vi "Draw_Grid.vi"(6 "Grid Color":u32(colorbox)=16711680, 8 "error in (no error)":errorcluster, 10 "Grid_Size":i32, 11 "Image_In":T1) -> (0 "error out":errorcluster, 3 "Image_Out":T1)   [LabVIEW 2020]
uses:
  <vilib>/vision/Image Controls.llb/IMAQ Image.ctl
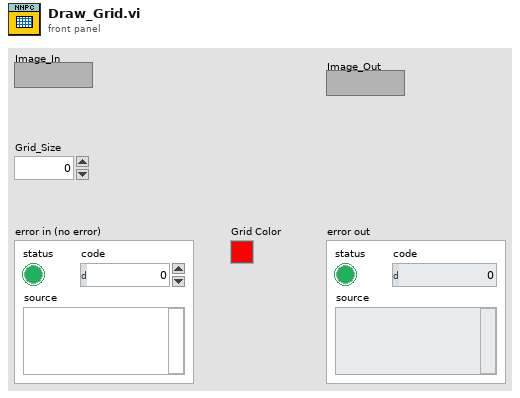
[diagram p1: front panel]
types:
  T1 = typedef "IMAQ Image.ctl" = refnum<image>
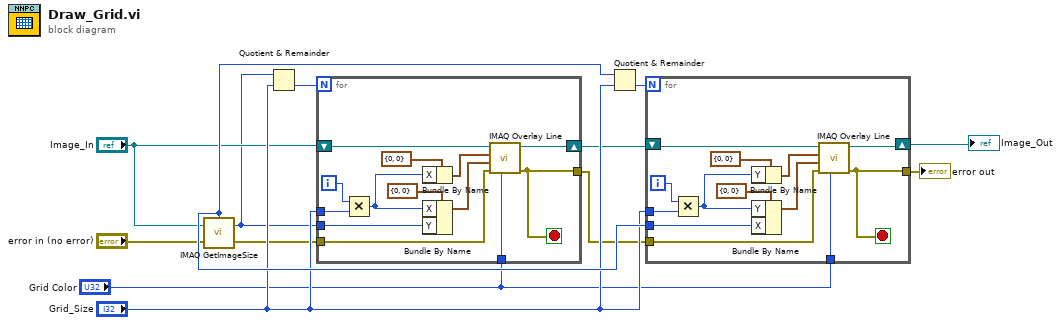
[diagram p0: block diagram]
diagram:
  n1 = call "IMAQ GetImageSize"("Image"="Image_In", "error in (no error)"="error in (no error)") -> ("Y Resolution"=w5:i32, "X Resolution"=w12:i32, "error out"=w4:errorcluster)  [unwired: 2 in]
  n2 = Quotient & Remainder(x=w5, y="Grid_Size") -> (floor(x/y)=w6:i32)  [unwired: 1 out]
  n3 = for {
    N: w6 -> [_]
    tunnel: w5 -> [w22]
    tunnel: w4 -> [w21]
    tunnel: "Grid_Size" -> [w20]
    tunnel: [w16] -> w9
    shift-right: [w15] -> w8
    shift-left: "Image_In" -> [w17]
    tunnel: "Grid Color" -> [w14]
    i -> [w19]
    stop <- w16 stop-if-true
    n4 = Multiply(x=w19, y=w20) -> (x*y=w18:i32)
    n5 = Bundle By Name(cluster=cluster{"X":i32, "Y":i32} {"X"=0, "Y"=0} ("Start Point"), "X"=w18) -> (w25:cluster{"X":i32, "Y":i32})
    n6 = Bundle By Name(cluster=cluster{"X":i32, "Y":i32} {"X"=0, "Y"=0} ("Start Point"), "X"=w18, "Y"=w22) -> (w23:cluster{"X":i32, "Y":i32})
    n7 = call "IMAQ Overlay Line"("Color"=w14, "error in (no error)"=w21, "End Point"=w23, "Start Point"=w25, "Image"=w17) -> ("error out"=w16:errorcluster, "Image Out"=w15:T1)  [unwired: 5 in]
  }
  n8 = Quotient & Remainder(x=w12, y="Grid_Size") -> (floor(x/y)=w10:i32)  [unwired: 1 out]
  n9 = for {
    N: w10 -> [_]
    tunnel: w12 -> [w29]
    tunnel: w9 -> [w35]
    tunnel: "Grid_Size" -> [w34]
    tunnel: [w30] -> w2
    shift-right: [w28] -> w13
    shift-left: w8 -> [w31]
    tunnel: "Grid Color" -> [w27]
    i -> [w33]
    stop <- w30 stop-if-true
    n10 = Multiply(x=w33, y=w34) -> (x*y=w32:i32)
    n11 = Bundle By Name(cluster=cluster{"X":i32, "Y":i32} {"X"=0, "Y"=0} ("Start Point"), "Y"=w32) -> (w38:cluster{"X":i32, "Y":i32})
    n12 = Bundle By Name(cluster=cluster{"X":i32, "Y":i32} {"X"=0, "Y"=0} ("Start Point"), "Y"=w32, "X"=w29) -> (w36:cluster{"X":i32, "Y":i32})
    n13 = call "IMAQ Overlay Line"("Color"=w27, "error in (no error)"=w35, "End Point"=w36, "Start Point"=w38, "Image"=w31) -> ("error out"=w30:errorcluster, "Image Out"=w28:T1)  [unwired: 5 in]
  }
  "Image_Out" <- w13
  "error out" <- w2
